vi "insertWidget.vi"(7 "index (-1)":i32=-1, 8 "Error In":errorcluster, 10 "widget":refnum<class "QWidget.lvclass">, 11 "QStackedWidget In":refnum<class "QStackedWidget.lvclass">) -> (0 "Error Out":errorcluster, 2 "Value":i32, 3 "QStackedWidget Out":refnum<class "QStackedWidget.lvclass">)   [LabVIEW 2014, in "QStackedWidget.lvclass"]
doc: "LabVIEW-specific documentation is not yet available. See <b>https://doc.qt.io/qt-5/qstackedwidget.html#insertWidget</b>"
uses:
  QStackedWidget.lvclass
  QWidget/QWidget.lvclass
  LQ Core/LQIdentity/LQIdentity.lvclass/LQIdentity.ctl
  LQ Core/LQ Core.lvlib
  LQ Core/LQIdentity/LQIdentity.lvclass
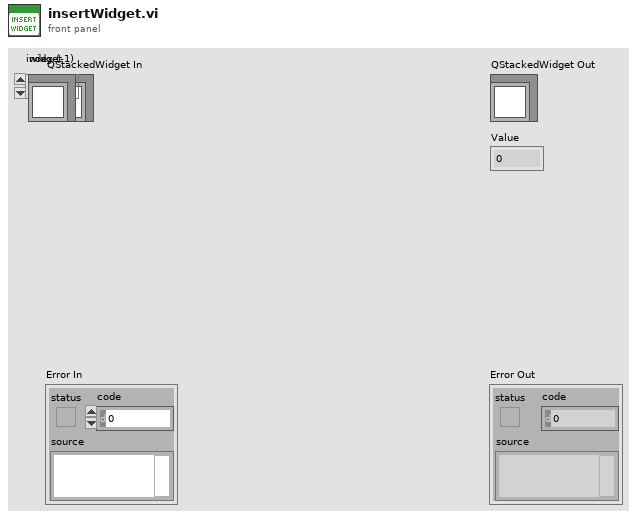
[diagram p1: front panel]
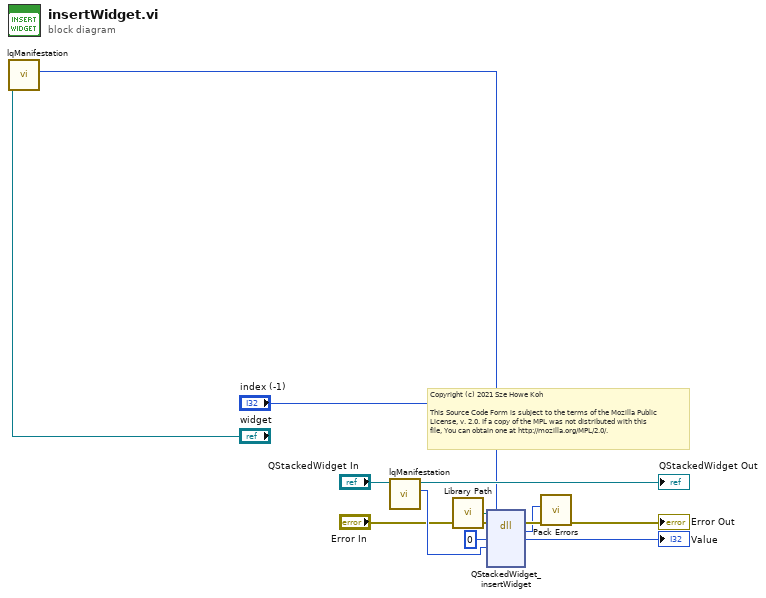
[diagram p0: block diagram]
diagram:
  # "Copyright (c) 2021 Sze Howe Koh\n\nThis Source Code Form is subject to the terms of the Mozilla Public\nLicense, v. 2.0. If a copy of the MPL was not distributed with this\nfile, You can obtain one at http://mozilla.org/MPL/2.0/."
  n1 = call "lqManifestation.vi"("LQIdentity in"="widget") -> ("Manifestation"=w1:u64)  [unwired: 9 in, 1 out]
  n2 = call "lqManifestation.vi"("LQIdentity in"="QStackedWidget In") -> ("Manifestation"=w8:u64, "LQIdentity out"=→"QStackedWidget Out":refnum<class "QStackedWidget.lvclass">)  [unwired: 9 in]
  n3 = call "Library Path.vi"() -> ("Library Path"=w9:path)
  n4 = dll-call lib="?" fn="QStackedWidget_insertWidget"(path in=w9, error in="Error In", "_retVal"=0 ("retVal"), "_instance"=w8, "index"="index (-1)", "widget"=w1) -> (error out=w6:errorcluster, w4:i32, "_retVal"=→"Value":i32)  [unwired: 4 in, 1 out]
  n5 = call "Pack Errors.vi"("Error In"=w6, "Error Code"=w4) -> ("Error Out"=→"Error Out":errorcluster)  [unwired: 9 in]
